vi "LabVIEW Read RF BIN without indicator and warmup.vi"(0 "file path":path=path "C:/Users/COCO/Desktop/TEMP.BIN") -> (4 "exec time":dbl)   [LabVIEW 2020]
uses:
  <vilib>/Analysis/2dsp.llb/Complex FFT.vi
  <vilib>/Analysis/NI_AALPro.lvlib
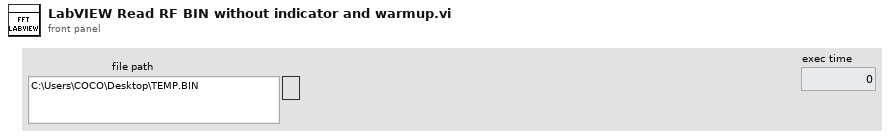
[diagram p1: front panel]
types:
  T1 = enum16{"open", "replace", "create", "open or create", "replace or create", "replace or create with confirmation"}
  T2 = enum16{"big-endian, network order", "native, host order", "little-endian"}
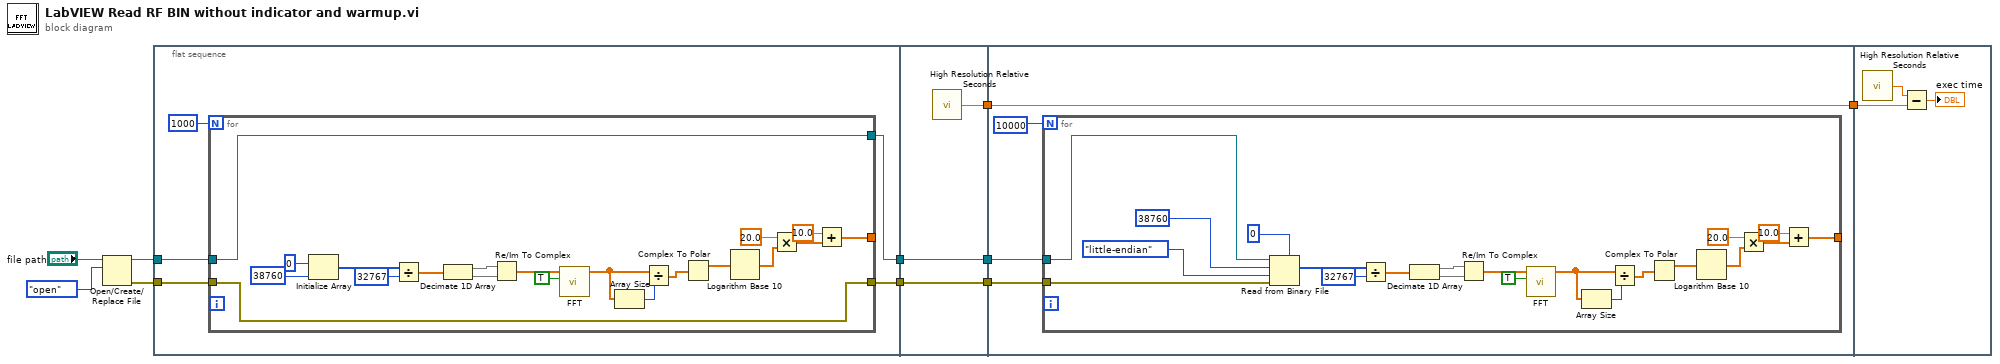
[diagram p0: block diagram]
diagram:
  n1 = Open/Create/Replace File(file path (use dialog)="file path", operation (0:open)=T1."open") -> (refnum out=w7:refnum<file>, error out=w8:errorcluster)  [unwired: 4 in, 1 out]
  n2 = flat-sequence {
    tunnel: w7 -> [w14]
    tunnel: w8 -> [w15]
    tunnel: [w13] -> w2
    tunnel: [w12] -> w1
    tunnel: [w38] -> w6
    tunnel: [w37] -> w5
    tunnel: [w36] -> w4
    tunnel: w2 -> [w37]
    tunnel: w1 -> [w38]
    tunnel: w6 -> [w42]
    tunnel: w5 -> [w41]
    tunnel: w4 -> [w39]
    tunnel: [w39] -> w3
    tunnel: w3 -> [w65]
    frame #0 {
      n3 = for {
        N: 1000 -> [_]
        tunnel: w15 -> [w16]
        tunnel: w14 -> [w20]
        tunnel: [w21] -> _
        tunnel: [w20] -> w13
        tunnel: [w16] -> w12
        n4 = Initialize Array(i16 0 ("Numeric"), 38760 ("count (1)")) -> (w17:i16[])
        n5 = Divide(x=w17, y=i16 32767 ("Numeric")) -> (x/y=w35:dbl[])
        n6 = Decimate 1D Array(w35) -> (w33:dbl[], w32:dbl[])
        n7 = Re/Im To Complex(1:w32, 2:w33) -> (0:w31:cdb[])
        n8 = call-poly <vilib>:"FFT.vi"("shift?"=TRUE, "X"=w31) -> ("FFT {X}"=w29:cdb[])  [unwired: 8 in, 1 out]
        n9 = Array Size(array=w29) -> (size(s)=w28:i32)
        n10 = Divide(x=w29, y=w28) -> (x/y=w30:cdb[])
        n11 = Complex To Polar(r * e^(i*theta)=w30) -> (r=w26:dbl[])  [unwired: 1 out]
        n12 = Logarithm Base 10(1:w26) -> (0:w25:dbl[])
        n13 = Multiply(x=20.0, y=w25) -> (x*y=w23:dbl[])
        n14 = Add(x=10.0, y=w23) -> (x+y=w21:dbl[])
      }
    }
    frame #1 {
      n15 = call <vilib>:"High Resolution Relative Seconds.vi"() -> ("relative seconds"=w36:dbl)
    }
    frame #2 {
      n16 = for {
        N: 10000 -> [_]
        tunnel: w42 -> [w63]
        tunnel: w41 -> [w62]
        tunnel: [w43] -> _
        n17 = Read from Binary File(5:i16 0 ("Numeric"), 8:w63, 9:T2."little-endian" ("byte order (0:big-endian, network order)"), 10:38760 ("count (1)"), 11:w62) -> (2:w58:i16[])  [unwired: 1 in, 3 out]
        n18 = Divide(x=w58, y=i16 32767 ("Numeric")) -> (x/y=w57:dbl[])
        n19 = Decimate 1D Array(w57) -> (w55:dbl[], w54:dbl[])
        n20 = Re/Im To Complex(1:w54, 2:w55) -> (0:w53:cdb[])
        n21 = call-poly <vilib>:"FFT.vi"("shift?"=TRUE, "X"=w53) -> ("FFT {X}"=w51:cdb[])  [unwired: 8 in, 1 out]
        n22 = Array Size(array=w51) -> (size(s)=w50:i32)
        n23 = Divide(x=w51, y=w50) -> (x/y=w52:cdb[])
        n24 = Complex To Polar(r * e^(i*theta)=w52) -> (r=w48:dbl[])  [unwired: 1 out]
        n25 = Logarithm Base 10(1:w48) -> (0:w47:dbl[])
        n26 = Multiply(x=20.0, y=w47) -> (x*y=w45:dbl[])
        n27 = Add(x=10.0, y=w45) -> (x+y=w43:dbl[])
      }
    }
    frame #3 {
      n28 = call <vilib>:"High Resolution Relative Seconds.vi"() -> ("relative seconds"=w66:dbl)
      n29 = Subtract(x=w66, y=w65) -> (x-y=→"exec time":dbl)
    }
  }
